vi "Request Data JSON.vi"(8 "error in (no error)":errorcluster, 11 "SetSceneItemEnabled in":refnum<class "SetSceneItemEnabled.lvclass">) -> (0 "error out":errorcluster, 2 "Request Data JSON":string, 3 "SetSceneItemEnabled out":refnum<class "SetSceneItemEnabled.lvclass">)   [LabVIEW 2022 SP3, in "obs-websocket-lv.lvlib" / "SetSceneItemEnabled.lvclass"]
uses:
  SetSceneItemEnabled.lvclass
  SetSceneItemEnabled.lvclass/SetSceneItemEnabled.ctl
  <vilib>/IlluminatedG/lv-web-crypto/lv-json/JSON/JSON.lvlib
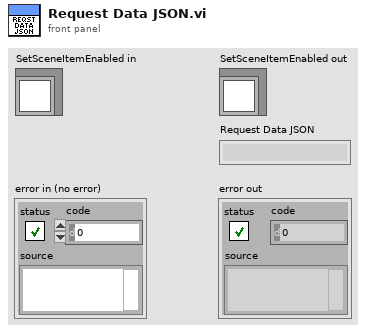
[diagram p1: front panel]
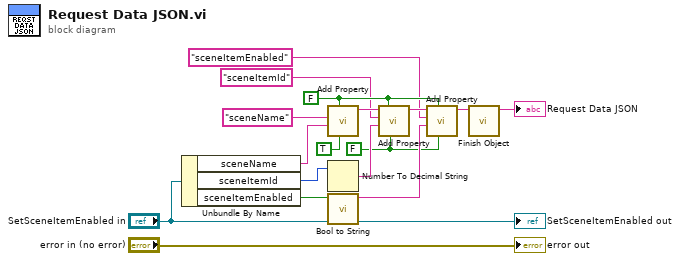
[diagram p0: block diagram]
diagram:
  w1 = FALSE ("String?")
  w6 = FALSE ("Include Empty?")
  n1 = Unbundle By Name("SetSceneItemEnabled in") -> ("sceneName"=w13:string, "sceneItemId"=w15:i32, "sceneItemEnabled"=w14:bool)
  n2 = call <vilib>:"Add Property.vi"("String?"=TRUE, "Include Empty?"=w6, "Value"=w13, "Property Name"="sceneName") -> ("String out"=w10:string)  [unwired: 7 in]
  n3 = Number To Decimal String(number=w15) -> (decimal integer string=w9:string)  [unwired: 1 in]
  n4 = call <vilib>:"Bool to String.vi"("Boolean"=w14) -> ("Value"=w7:string)  [unwired: 10 in]
  n5 = call <vilib>:"Add Property.vi"("String?"=w1, "Include Empty?"=w6, "Value"=w9, "Property Name"="sceneItemId", "String In"=w10) -> ("String out"=w8:string)  [unwired: 6 in]
  n6 = call <vilib>:"Add Property.vi"("String?"=w1, "Include Empty?"=w6, "Value"=w7, "Property Name"="sceneItemEnabled", "String In"=w8) -> ("String out"=w3:string)  [unwired: 6 in]
  n7 = call <vilib>:"Finish Object.vi"("String In"=w3) -> ("String out"=→"Request Data JSON":string)  [unwired: 10 in]
  "error out" <- "error in (no error)"
  "SetSceneItemEnabled out" <- "SetSceneItemEnabled in"
